vi "sr830 dsp lock in.vi"(8 "error in (no error)":errorcluster, 10 "Parameter (1: X)":u16(ring)=4 items=["X"=1, "Y"=2, "R"=3, "Theta"=4, "Channel 1"=5, "Channel 2"=6, "Aux In 1"=7, "Aux In 2"=8, "Aux In 3"=9, "Aux In 4"=10], 11 "VISA resource name":refnum<visa-resource-name>="GPIB0::8::INSTR") -> (0 "error out":errorcluster, 2 "Datos Lokin String":string, 3 "Medición":dbl)   [LabVIEW 2017]
uses:
  <instrlib>/Stanford Research 830/Public/Data/Read (1 Parameter).vi
  <instrlib>/Stanford Research 830/Stanford Research 830.lvlib
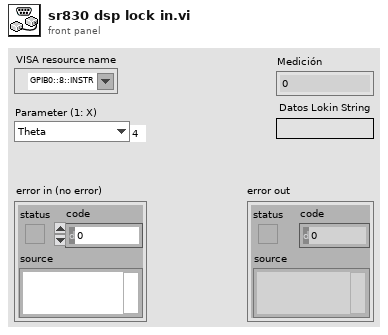
[diagram p1: front panel]
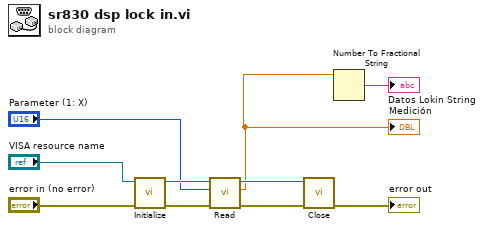
[diagram p0: block diagram]
diagram:
  n1 = call <instrlib>:"Initialize.vi"("error in (no error)"="error in (no error)", "VISA resource name"="VISA resource name") -> ("error out"=w9:errorcluster, "VISA resource name out"=w10:refnum<visa-resource-name>)  [unwired: 8 in]
  n2 = call-poly <instrlib>:"Read.vi"("error in (no error)"=w9, "Parameter (1: X)"="Parameter (1: X)", "VISA resource name"=w10) -> ("error out"=w6:errorcluster, "Measurement"=w2:dbl, "VISA resource name out"=w7:refnum<visa-resource-name>)  [unwired: 6 in]
  "Medición" <- w2
  n3 = call <instrlib>:"Close.vi"("error in (no error)"=w6, "VISA resource name"=w7) -> ("error out"=→"error out":errorcluster)  [unwired: 9 in]
  n4 = Number To Fractional String(number=w2) -> (F-format string=→"Datos Lokin String":string)  [unwired: 3 in]
